vi "DesignPatterns_DrawNodesAndLinks.vi"(0 "GraphIn":refnum<class "Graph.lvclass">, 1 "Graphics":refnum<class "Graphics.lvclass">, 2 "Grid":refnum<class "Grid.lvclass">, 3 "Nodes":T1[](array[typedef]), 4 "Links":T3[](array[typedef]), 5 "error in (no error)":errorcluster, 6 "Y-Offset":i32, 7 "NodeIndexies":i32[](array[numeric]), 8 "X-Offset":i32) -> (14 "GraphOut":refnum<class "Graph.lvclass">, 16 "NodesCreated/Modified":refnum<class "AbstractNode.lvclass">[](array[class]), 19 "error out":errorcluster)   [LabVIEW 2020]
uses:
  <resource>/Framework/Providers/Open_GDS/UML/Grid_class/Grid.lvclass
  <resource>/Framework/Providers/Open_GDS/UML/Graphics_class/Graphics.lvclass
  <resource>/Framework/Providers/Open_GDS/UML/Graph_class/Graph.lvclass
  <resource>/Framework/Providers/Open_GDS/UML/DesignPattern/SubVIs/DesignPatterns_Link.ctl
  <resource>/Framework/Providers/Open_GDS/UML/DesignPattern/SubVIs/DesignPatterns_LinkType.ctl
  <resource>/Framework/Providers/Open_GDS/UML/DesignPattern/SubVIs/DesignPatterns_Node.ctl
  <resource>/Framework/Providers/Open_GDS/UML/DesignPattern/SubVIs/DesignPatterns_NodeType.ctl
  <resource>/Framework/Providers/Open_GDS/UML/AbstractNode_class/AbstractNode.lvclass
  <resource>/Framework/Providers/Open_GDS/UML/General/Point/Point Point2D.ctl
  <resource>/Framework/Providers/Open_GDS/UML/DesignPattern/SubVIs/DesignPatterns_ClassNodeData.ctl
  <resource>/Framework/Providers/Open_GDS/UML/DesignPattern/SubVIs/DesignPatterns_Attribute.ctl
  <resource>/Framework/Providers/Open_GDS/UML/DesignPattern/SubVIs/DesignPatterns_Method.ctl
  <resource>/Framework/Providers/Open_GDS/UML/DesignPattern/SubVIs/DesignPatterns_NoteNodeData.ctl
  <resource>/Framework/Providers/Open_GDS/UML/DesignPattern/SubVIs/DesignPatterns_NoteLink.ctl
  <resource>/Framework/Providers/Open_GDS/UML/Graph_class/AddItemsToGraph_Edges.ctl
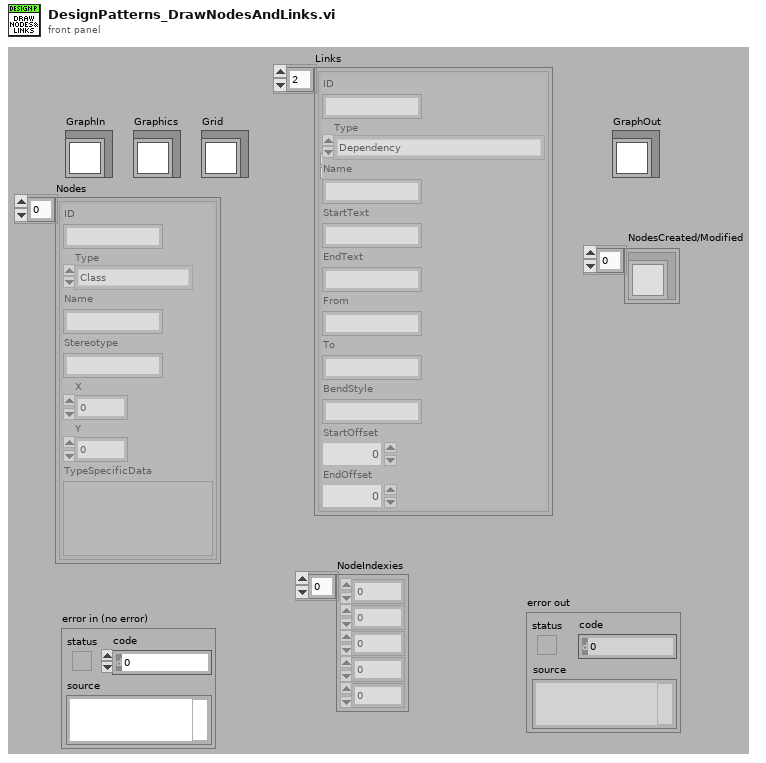
[diagram p1: front panel]
types:
  T1 = typedef "DesignPatterns_Node.ctl" = cluster{"ID":string, "Type":T2, "Name":string, "Stereotype":string, "X":i32, "Y":i32, "TypeSpecificData":variant}
  T2 = typedef "DesignPatterns_NodeType.ctl" = enum16{"Class", "Interface", "Note", "Package"}
  T3 = typedef "DesignPatterns_Link.ctl" = cluster{"ID":string, "Type":T4, "Name":string, "StartText":string, "EndText":string, "From":string, "To":string, "BendStyle":string, "StartOffset":i32, "EndOffset":i32}
  T4 = typedef "DesignPatterns_LinkType.ctl" = enum16{"Dependency", "Inheritance", "Interface", "Association", "Aggregation", "CompositeAggregation"}
  T5 = typedef "Point Point2D.ctl" = cluster{"x":dbl, "y":dbl}
  T6 = cluster{"Text":string, "Point":T5, "Links":string[]}[]
  T7 = cluster{"Name":string, "Attributes":string, "Methods":string, "Point":T5, "Interface":bool}[]
  T8 = typedef "DesignPatterns_ClassNodeData.ctl" = cluster{"Description":string, "Attributes":T9[], "Methods":T10[]}
  T9 = typedef "DesignPatterns_Attribute.ctl" = cluster{"ID":string, "Name":string}
  T10 = typedef "DesignPatterns_Method.ctl" = cluster{"ID":string, "Name":string}
  T11 = cluster{"Name":string, "Attributes":string, "Methods":string, "Point":T5, "Interface":bool}
  T12 = cluster{"Text":string, "Point":T5, "Links":string[]}
  T13 = typedef "DesignPatterns_NoteNodeData.ctl" = cluster{"Text":string, "Links":T14[]}
  T14 = typedef "DesignPatterns_NoteLink.ctl" = cluster{"ID":string, "source":string}
  T15 = typedef "Graph.lvclass/AddItemsToGraph_Edges.ctl" = cluster{"Type":T4, "From":i32, "To":i32, "Name":string, "StartText":string, "EndText":string, "BendStyle":string, "StartOffset":i32, "EndOffset":i32}
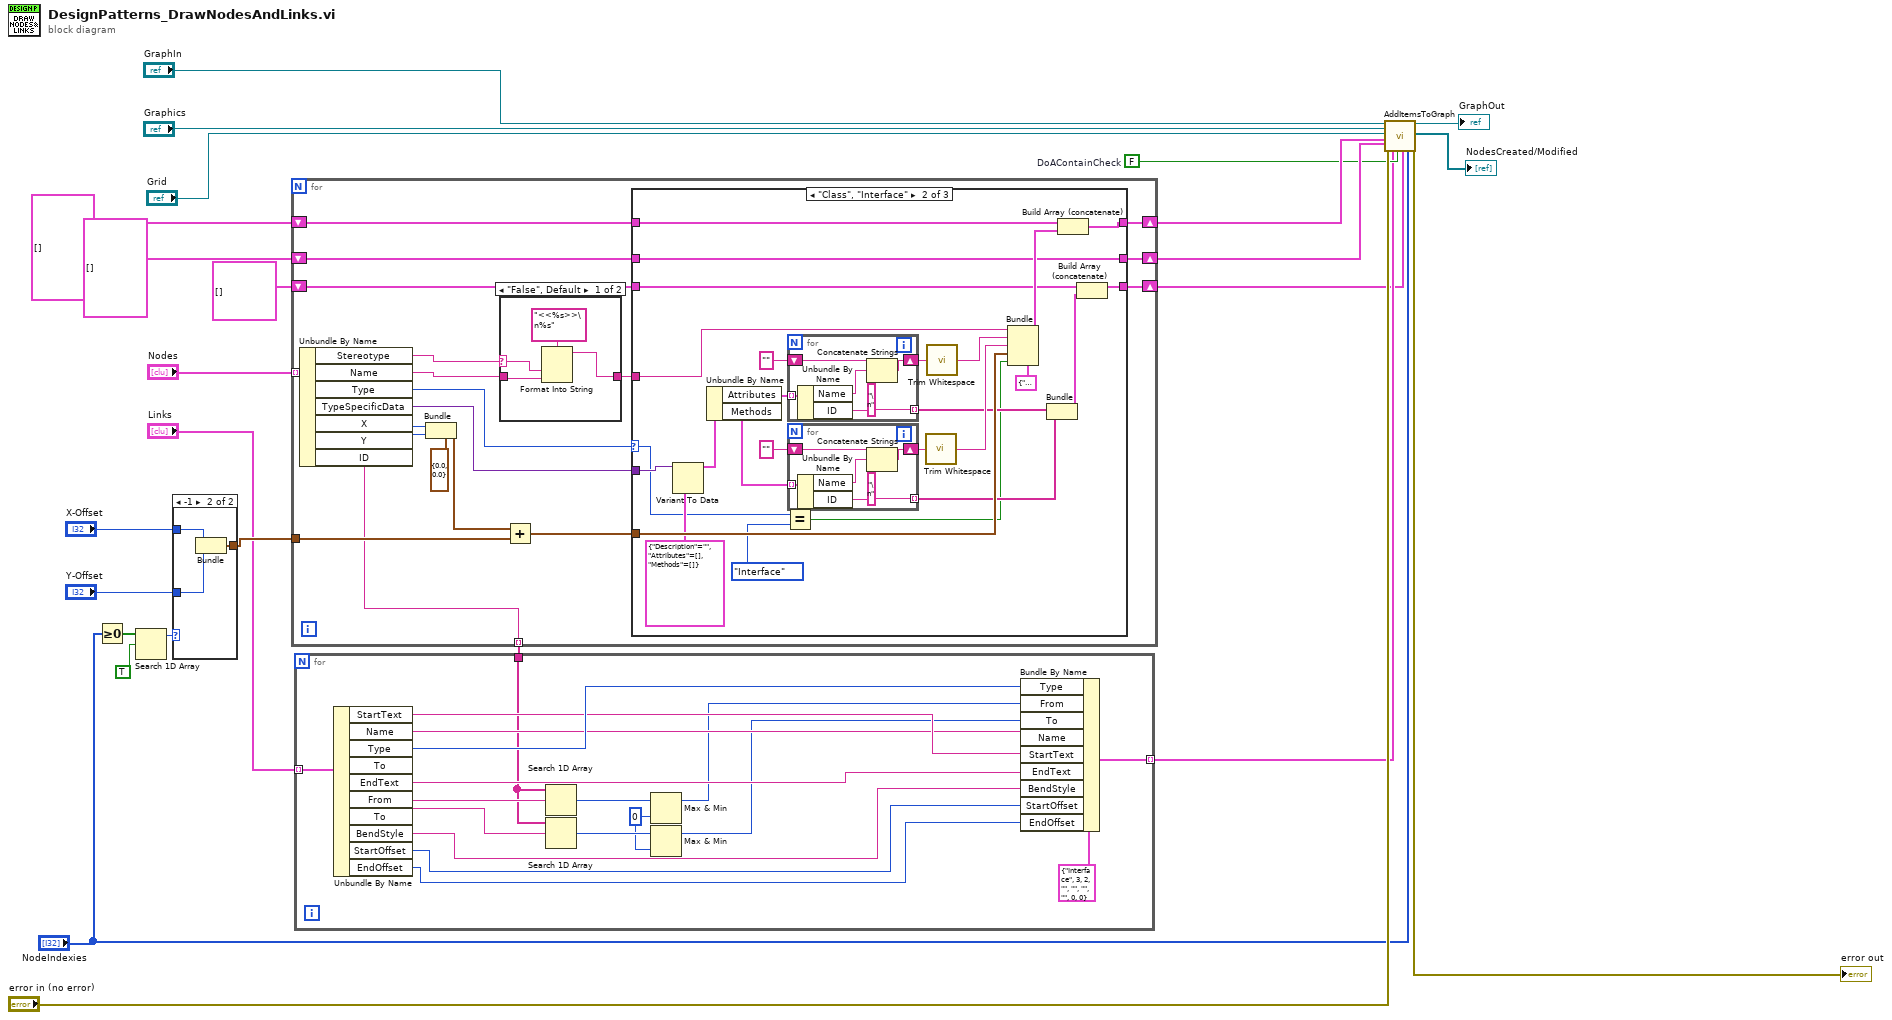
[diagram p0: block diagram]
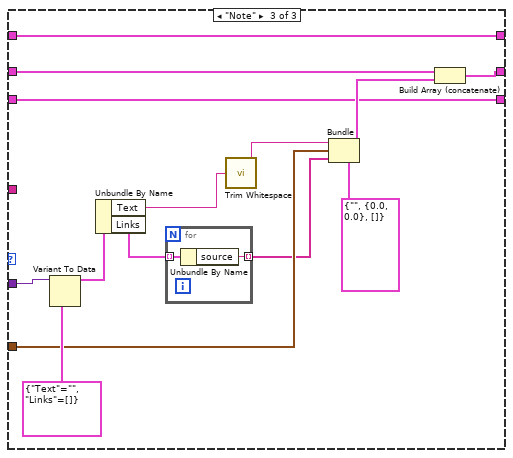
[diagram p4: hidden frame]
diagram:
  w13 = FALSE  # DoAContainCheck
  n1 = Greater Or Equal To 0?(x="NodeIndexies") -> (x >= 0?=w3:bool[])
  n2 = Search 1D Array(1D array=w3, element=TRUE) -> (index of element=w1:i32)  [unwired: 1 in]
  n3 = case shown="-1" w1 {
    tunnel: "X-Offset" -> [_ w28]
    tunnel: "Y-Offset" -> [_ w27]
    tunnel: [_ w26] -> w21
    frame Default {
    }
    frame -1 {
      n4 = Bundle("X-Offset"=w28, "Y-Offset"=w27) -> (w26:cluster{"X-Offset":i32, "Y-Offset":i32})  [unwired: 1 in]
    }
  }
  n5 = for {
    tunnel: "Nodes" -> [w47] mode=indexing
    shift-right: [w35] -> w20
    shift-left: T7 [] -> [w36]
    tunnel: w21 -> [w38]
    shift-right: [w33] -> w14
    shift-left: T6 [] ("NotNodes") -> [w32]
    tunnel: [w31] -> w9 mode=indexing
    shift-right: [w30] -> w6
    shift-left: cluster{string[], string[]}[] [] -> [w29]
    n6 = Unbundle By Name(w47) -> ("Stereotype"=w46:string, "Name"=w45:string, "Type"=w44:T2, "TypeSpecificData"=w34:variant, "X"=w42:i32, "Y"=w41:i32, "ID"=w31:string)
    n7 = Bundle(cluster=T5 {"x"=0.0, "y"=0.0} ("Point"), "x"=w42, "y"=w41) -> (w40:T5)
    n8 = case shown="\"False\", Default" w46 {
      selector: w46 -> [w107 _]
      tunnel: w45 -> [w106 w109]
      tunnel: [w105 w109] -> w43
      frame "False", Default {
        n9 = Format Into String(format string="<<%s>>\n%s", w107, w106) -> (resulting string=w105:string)  [unwired: 2 in, 1 out]
      }
      frame "" {
      }
    }
    n10 = Add(x=w40, y=w38) -> (x+y=w37:T5)
    n11 = case shown="\"Class\", \"Interface\"" w44 {
      selector: w44 -> [_ w53 _]
      tunnel: w43 -> [_ w75 _]
      tunnel: w37 -> [_ w74 w95]
      tunnel: w36 -> [w50 w73 w92]
      tunnel: [w50 w71 w92] -> w35
      tunnel: w34 -> [_ w70 w102]
      tunnel: w32 -> [w49 w59 w97]
      tunnel: [w49 w59 w98] -> w33
      tunnel: [w48 w58 w89] -> w30
      tunnel: w29 -> [w48 w57 w89]
      frame Default {
      }
      frame "Class", "Interface" {
        n12 = Variant To Data(type=T8 {"Description"="", "Attributes"=[], "Methods"=[]}, Variant=w70) -> (data=w68:T8)  [unwired: 1 in, 1 out]
        n13 = Unbundle By Name(w68) -> ("Attributes"=w67:T9[], "Methods"=w64:T10[])
        n14 = Equal?(x=w53, y=DesignPatterns_NodeType."Interface") -> (x = y?=w51:bool)
        n15 = for {
          tunnel: w67 -> [w88] mode=indexing
          shift-right: [w86] -> w63
          shift-left: "" -> [w87]
          tunnel: [w83] -> w56 mode=indexing
          n16 = Unbundle By Name(w88) -> ("Name"=w85:string, "ID"=w83:string)
          n17 = Concatenate Strings(w87, w85, "\n" ("string")) -> (w86:string)
        }
        n18 = for {
          tunnel: w64 -> [w82] mode=indexing
          shift-right: [w80] -> w62
          shift-left: "" -> [w81]
          tunnel: [w77] -> w55 mode=indexing
          n19 = Unbundle By Name(w82) -> ("Name"=w79:string, "ID"=w77:string)
          n20 = Concatenate Strings(w81, w79, "\n" ("string")) -> (w80:string)
        }
        n21 = call <vilib>:"Trim Whitespace.vi"("string"=w62) -> ("trimmed string"=w60:string)  [unwired: 1 in]
        n22 = call <vilib>:"Trim Whitespace.vi"("string"=w63) -> ("trimmed string"=w61:string)  [unwired: 1 in]
        n23 = Bundle(cluster=T11 {"Name"="", "Attributes"="", "Methods"="", "Point"={"x"=0.0, "y"=0.0}, "Interface"=FALSE} ("Node"), "Name"=w75, "Attributes"=w61, "Methods"=w60, "Point"=w74, "Interface"=w51) -> (w72:T11)
        n24 = Bundle(w56, w55) -> (w54:cluster{string[], string[]})  [unwired: 1 in]
        n25 = Build Array (concatenate)(w73, w72) -> (w71:T7)
        n26 = Build Array (concatenate)(w57, w54) -> (w58:cluster{string[], string[]}[])
      }
      frame "Note" {
        n27 = Variant To Data(type=T13 {"Text"="", "Links"=[]}, Variant=w102) -> (data=w100:T13)  [unwired: 1 in, 1 out]
        n28 = Unbundle By Name(w100) -> ("Text"=w99:string, "Links"=w91:T14[])
        n29 = for {
          tunnel: w91 -> [w104] mode=indexing
          tunnel: [w103] -> w90 mode=indexing
          n30 = Unbundle By Name(w104) -> ("source"=w103:string)
        }
        n31 = call <vilib>:"Trim Whitespace.vi"("string"=w99) -> ("trimmed string"=w94:string)  [unwired: 1 in]
        n32 = Bundle(cluster=T12 {"Text"="", "Point"={"x"=0.0, "y"=0.0}, "Links"=[]} ("Note"), "Text"=w94, "Point"=w95, "Links"=w90) -> (w93:T12)
        n33 = Build Array (concatenate)(w97, w93) -> (w98:T6)
      }
    }
  }
  n34 = for {
    tunnel: "Links" -> [w127] mode=indexing
    tunnel: [w126] -> w10 mode=indexing
    tunnel: w9 -> [w120]
    w114 = 0 ("y")
    n35 = Unbundle By Name(w127) -> ("StartText"=w123:string, "Name"=w122:string, "Type"=w125:T4, "EndText"=w124:string, "From"=w121:string, "To"=w119:string, "BendStyle"=w112:string, "StartOffset"=w111:i32, "EndOffset"=w110:i32)  [unwired: 1 out]
    n36 = Search 1D Array(1D array=w120, element=w121) -> (index of element=w118:i32)  [unwired: 1 in]
    n37 = Search 1D Array(1D array=w120, element=w119) -> (index of element=w116:i32)  [unwired: 1 in]
    n38 = Max & Min(x=w118, y=w114) -> (max(x,y)=w117:i32)  [unwired: 1 out]
    n39 = Max & Min(x=w116, y=w114) -> (max(x,y)=w115:i32)  [unwired: 1 out]
    n40 = Bundle By Name(cluster=T15 {"Type"=enum."Interface", "From"=3, "To"=2, "Name"="", "StartText"="", "EndText"="", "BendStyle"="", "StartOffset"=0, "EndOffset"=0} ("Cluster"), "Type"=w125, "From"=w117, "To"=w115, "Name"=w122, "StartText"=w123, "EndText"=w124, "BendStyle"=w112, "StartOffset"=w111, "EndOffset"=w110) -> (w126:T15)
  }
  n41 = call <resource>:"AddItemsToGraph.vi"("GraphIn"="GraphIn", "graphics"="Graphics", "grid"="Grid", "ClassNodes"=w20, "NoteNodes"=w14, "error in (no error)"="error in (no error)", "Links"=w10, "DoAContainCheck"=w13, "ClassNodesAtt/MethodIDs"=w6, "NodeIndexiesToOnlyUpdate"="NodeIndexies") -> ("GraphOut"=→"GraphOut":refnum<class "Graph.lvclass">, "NodesCreated/Modified"=→"NodesCreated/Modified":refnum<class "AbstractNode.lvclass">[], "error out"=→"error out":errorcluster)  [unwired: 7 in]
